vi "Airy Functions.vi"(7 "x":dbl format="%.2f") -> (2 "Bi(x)":dbl format="%.2f", 3 "Ai(x)":dbl format="%.2f")   [LabVIEW 2014, in "NI_Gmath.lvlib"]
doc: "Computes the Airy functions <B>Ai(x)</B> and <B>Bi(x)</B>."
uses:
  NI_Gmath.lvlib
  lvanlys.dll
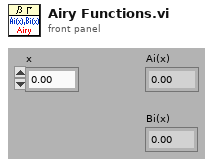
[diagram p1: front panel]
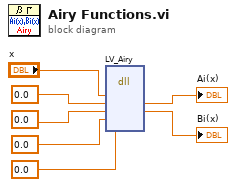
[diagram p0: block diagram]
diagram:
  n1 = dll-call lib="C:/Program Files (x86)/National Instruments/LabVIEW 2014/resource/lvanlys.*" fn="LV_Airy"("x"="x", "Ai"=0.0, "Bi"=0.0 ("Ai"), "dAi"=0.0 ("Ai"), "dBi"=0.0 ("Ai")) -> ("Ai"=→"Ai(x)":dbl, "Bi"=→"Bi(x)":dbl)  [unwired: 7 in, 2 out]
